vi "teste-fit-1.vi"() -> ()   [LabVIEW 2014]
uses:
  <vilib>/Analysis/NI_AALPro.lvlib
panel:
  out "XY Graph 3":cluster{i32[], "Array":dbl[]}[](graph)
  out "intercept":dbl
  out "slope":dbl
  out "XY Graph 2":cluster{i32[], "Best Linear Fit":dbl[]}[](graph)
  out "XY Graph":cluster{i32[], dbl[]}[](graph)
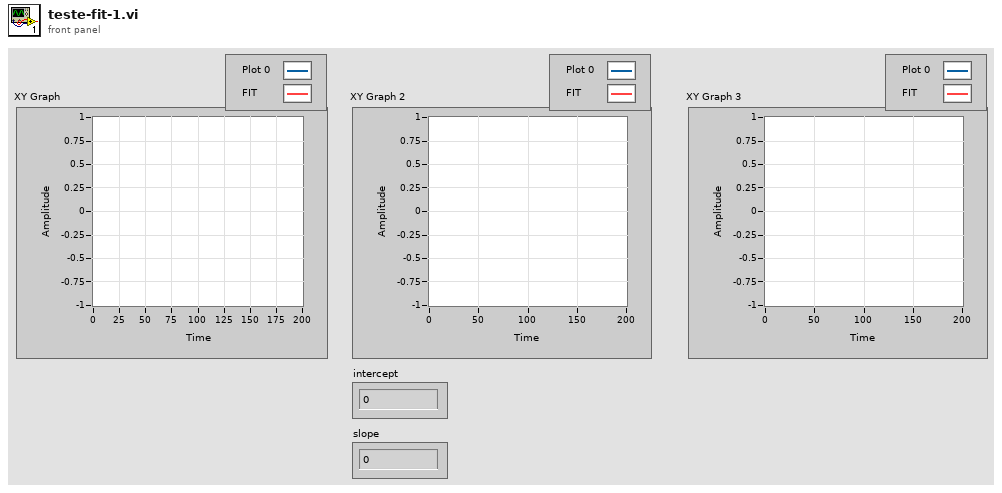
[diagram p1: front panel]
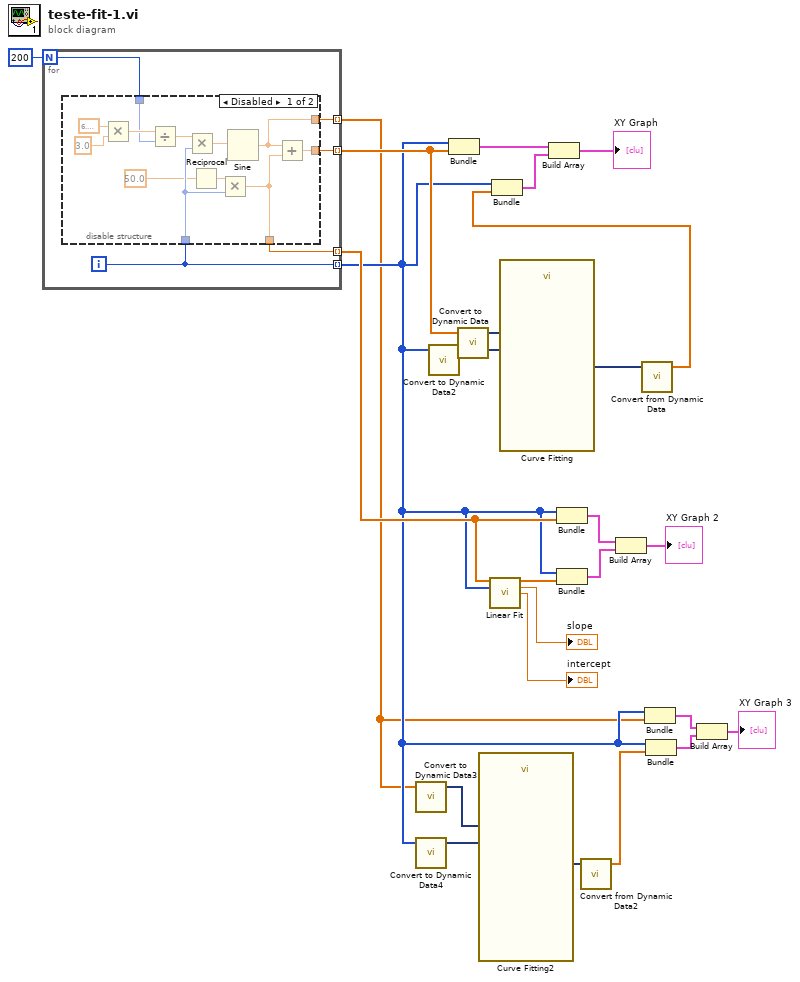
[diagram p0: block diagram]
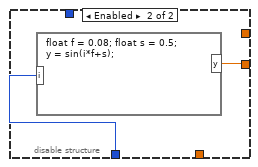
[diagram p2: hidden frame]
diagram:
  n1 = for {
    N: 200 -> [w30]
    tunnel: [w29] -> w9 mode=indexing
    tunnel: [w28] -> w5 mode=indexing
    tunnel: [w27] -> w10 mode=indexing
    tunnel: [w26] -> w4 mode=indexing
    i -> [w28]
    n2 = disable-structure shown="Disabled" {
      disable-tunnel: w30 -> [w37 _]
      disable-tunnel: [w36 w43] -> w29
      disable-tunnel: w28 -> [w34 w44]
      disable-tunnel: [w32 _] -> w27
      disable-tunnel: [w31 _] -> w26
      frame Disabled {
        n3 = Multiply(x=6.283185307179586, y=3.0) -> (x*y=w40:dbl)
        n4 = Divide(x=w40, y=w37) -> (x/y=w39:dbl)
        n5 = Multiply(x=w39, y=w34) -> (x*y=w38:dbl)
        n6 = Reciprocal(x=50.0) -> (1/x=w35:dbl)
        n7 = Multiply(x=w35, y=w34) -> (x*y=w32:dbl)
        n8 = Sine(x=w38) -> (sin(x)=w31:dbl)
        n9 = Add(x=w31, y=w32) -> (x+y=w36:dbl)
      }
      frame Enabled {
        n10 = formula code="float f = 0.08; float s = 0.5;\ny = sin(i*f+s);"("i"=w44) -> ("y"=w43:dbl)
      }
    }
  }
  n11 = call "Convert to Dynamic Data3"("Array"=w4) -> ("Dynamic Data Type"=w12:dynamicdata)  [unwired: 3 in]
  n12 = call "Convert to Dynamic Data4"("Array"=w5) -> ("Dynamic Data Type"=w11:dynamicdata)  [unwired: 3 in]
  n13 = call "Convert to Dynamic Data2"("Array"=w5) -> ("Dynamic Data Type"=w23:dynamicdata)  [unwired: 3 in]
  n14 = Bundle(w5, w9) -> (w22:cluster{i32[], dbl[]})  [unwired: 1 in]
  n15 = call "Convert to Dynamic Data"("Array"=w9) -> ("Dynamic Data Type"=w24:dynamicdata)  [unwired: 3 in]
  n16 = call "Curve Fitting2"("Locations"=w11, "Signals"=w12) -> ("best fit"=w8:dynamicdata)  [unwired: 5 in, 4 out]
  n17 = call <vilib>:"Linear Fit.vi"("Y"=w10, "X"=w5) -> ("Best Linear Fit"=w17:dbl[], "slope"=→"slope":dbl, "intercept"=→"intercept":dbl)  [unwired: 9 in, 2 out]
  n18 = call "Curve Fitting"("Locations"=w23, "Signals"=w24) -> ("best fit"=w21:dynamicdata)  [unwired: 5 in, 4 out]
  n19 = Bundle(w5, w10) -> (w16:cluster{i32[], dbl[]})  [unwired: 1 in]
  n20 = Bundle(w5, "Best Linear Fit"=w17) -> (w6:cluster{i32[], "Best Linear Fit":dbl[]})  [unwired: 1 in]
  n21 = call "Convert from Dynamic Data2"("Dynamic Data Type"=w8) -> ("Array"=w7:dbl[])  [unwired: 3 in]
  n22 = Build Array(w16, w6) -> (→"XY Graph 2":cluster{i32[], "Best Linear Fit":dbl[]}[])
  n23 = call "Convert from Dynamic Data"("Dynamic Data Type"=w21) -> ("Array"=w20:dbl[])  [unwired: 3 in]
  n24 = Bundle(w5, "Array"=w20) -> (w19:cluster{i32[], "Array":dbl[]})  [unwired: 1 in]
  n25 = Build Array(w22, w19) -> (→"XY Graph":cluster{i32[], "Array":dbl[]}[])
  n26 = Bundle(w5, w4) -> (w3:cluster{i32[], dbl[]})  [unwired: 1 in]
  n27 = Bundle(w5, "Array"=w7) -> (w2:cluster{i32[], "Array":dbl[]})  [unwired: 1 in]
  n28 = Build Array(w3, w2) -> (→"XY Graph 3":cluster{i32[], "Array":dbl[]}[])
